vi "Cryo Magnet (SubVI) I.vi"(0 "Instrument parameters":T1, 3 "Max Rate":dbl=0.5 format="%#_13g", 5 "Target":dbl, 7 "Present value":dbl, 9 "Sweep rate":dbl, 11 "error in (no error)":errorcluster, 12 "Timeout (s)":u16, 14 "Default Rate":dbl=0.25 format="%#_13g") -> (4 "Instrument parameters out":T1, 6 "Last field":dbl, 15 "error out":errorcluster)   [LabVIEW 2016]
uses:
  TYPE DEFS/S2DS_Instrument parameters.ctl
  Cryo.lvlib
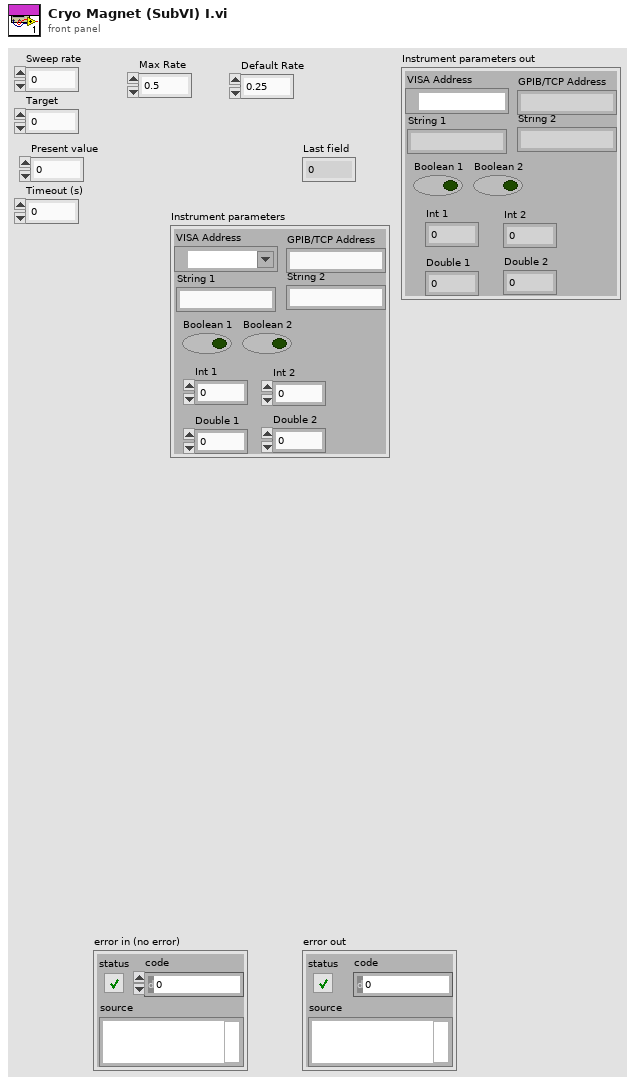
[diagram p1: front panel]
types:
  T1 = typedef "S2DS_Instrument parameters.ctl" = cluster{"VISA Address":refnum<visa-resource-name>, "GPIB/TCP Address":string, "String 1":string, "String 2":string, "Boolean 1":bool, "Boolean 2":bool, "Int 1":i32, "Int 2":i32, "Double 1":dbl, "Double 2":dbl}
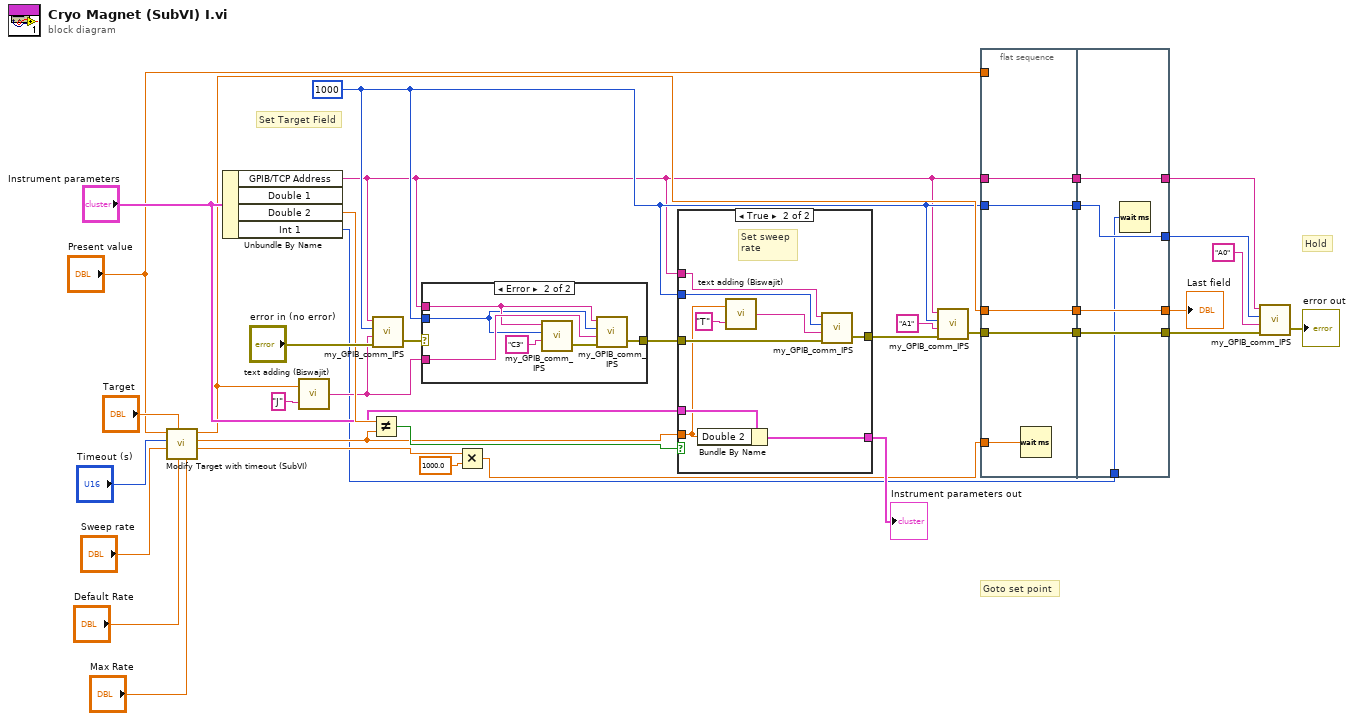
[diagram p0: block diagram]
diagram:
  w6 = u32 1000 ("Timeout (ms)")
  # "Goto set point"
  # "Set Target Field"
  # "Hold"
  n1 = call "Modify Target with timeout (SubVI).vi"("Max Rate"="Max Rate", "Default Rate"="Default Rate", "Target in"="Target", "Sweep rate in"="Sweep rate", "Timeout (s) in"="Timeout (s)", "Present value"="Present value") -> ("Timeout (s) out"=w9:dbl, "Sweep rate out"=w12:dbl, "Target out"=w14:dbl)  [unwired: 3 in]
  n2 = Unbundle By Name("Instrument parameters") -> ("GPIB/TCP Address"=w4:string, "Double 2"=w17:dbl, "Int 1"=w2:i32)  [unwired: 1 out]
  n3 = call "text adding (Biswajit).vi"("string"="J", "number"=w14) -> ("String"=w5:string)
  n4 = Not Equal?(x=w17, y=w12) -> (x != y?=w16:bool)
  n5 = call "my_GPIB_comm_IPS.vi"("error in"="error in (no error)", "Command"=w5, "Timeout (ms)"=w6, "GPIB address"=w4) -> ("error out"=w8:errorcluster)  [unwired: 1 out]
  n6 = case shown="Error" w8 {
    selector: w8 -> [w37 _]
    tunnel: [w37 w38] -> w7
    tunnel: w4 -> [_ w40]
    tunnel: w6 -> [_ w39]
    tunnel: w5 -> [_ w41]
    frame No Error {
    }
    frame Error {
      n7 = call "my_GPIB_comm_IPS.vi"("Command"="C3", "Timeout (ms)"=w39, "GPIB address"=w40) -> ("error out"=w42:errorcluster)  [unwired: 1 in, 1 out]
      n8 = call "my_GPIB_comm_IPS.vi"("error in"=w42, "Command"=w41, "Timeout (ms)"=w39, "GPIB address"=w40) -> ("error out"=w38:errorcluster)  [unwired: 1 out]
    }
  }
  n9 = Multiply(x=w9, y=1000.0) -> (x*y=w1:dbl)
  n10 = case shown="True" w16 {
    tunnel: w4 -> [_ w54]
    tunnel: w7 -> [w45 w53]
    tunnel: [w45 w52] -> w22
    tunnel: w12 -> [_ w48]
    tunnel: "Instrument parameters" -> [w44 w49]
    tunnel: w6 -> [_ w47]
    tunnel: [w44 w46] -> w3
    frame False {
    }
    frame True {
      # "Set sweep \nrate"
      n11 = Bundle By Name(cluster=w49, "Double 2"=w48) -> (w46:T1)
      n12 = call "text adding (Biswajit).vi"("string"="T", "number"=w48) -> ("String"=w51:string)
      n13 = call "my_GPIB_comm_IPS.vi"("error in"=w53, "Command"=w51, "Timeout (ms)"=w47, "GPIB address"=w54) -> ("error out"=w52:errorcluster)  [unwired: 1 out]
    }
  }
  "Instrument parameters out" <- w3
  n14 = call "my_GPIB_comm_IPS.vi"("error in"=w22, "Command"="A1", "Timeout (ms)"=w6, "GPIB address"=w4) -> ("error out"=w25:errorcluster)  [unwired: 1 out]
  n15 = flat-sequence {
    tunnel: w4 -> [w59]
    tunnel: w25 -> [w58]
    tunnel: w14 -> [w56]
    tunnel: w6 -> [w57]
    tunnel: [w59] -> w30
    tunnel: [w58] -> w29
    tunnel: [w56] -> w28
    tunnel: [w57] -> w27
    tunnel: "Present value" -> [_]
    tunnel: w1 -> [w55]
    tunnel: [w62] -> w24
    tunnel: [w64] -> w35
    tunnel: [w63] -> w26
    tunnel: w30 -> [w63]
    tunnel: w29 -> [w61]
    tunnel: w28 -> [w64]
    tunnel: w27 -> [w62]
    tunnel: [w61] -> w19
    tunnel: w2 -> [w60]
    frame #0 {
      n16 = Wait (ms)(milliseconds to wait=w55) -> ()  [unwired: 1 out]
    }
    frame #1 {
      n17 = Wait (ms)(milliseconds to wait=w60) -> ()  [unwired: 1 out]
    }
  }
  n18 = call "my_GPIB_comm_IPS.vi"("error in"=w19, "Command"="A0", "Timeout (ms)"=w24, "GPIB address"=w26) -> ("error out"=→"error out":errorcluster)  [unwired: 1 out]
  "Last field" <- w35
